vi "mein_sensor.vi"(11 "Position":dbl format="%_3g") -> (3 "Sensorsignal":dbl format="%_3g")   [LabVIEW 2019]
panel:
  out "R_aussen":bool
  out "R":bool
  out "L":bool
  out "L_aussen":bool
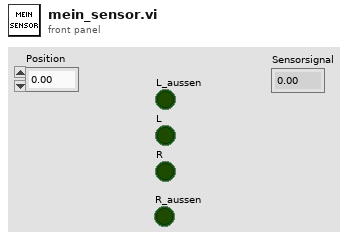
[diagram p1: front panel]
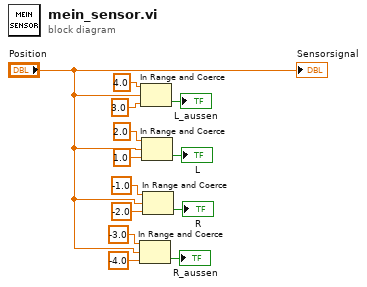
[diagram p0: block diagram]
diagram:
  n1 = In Range and Coerce(upper limit=-3.0, x="Position", lower limit=-4.0) -> (In Range?=→"R_aussen":bool)  [unwired: 1 out]
  n2 = In Range and Coerce(upper limit=4.0, x="Position", lower limit=3.0) -> (In Range?=→"L_aussen":bool)  [unwired: 1 out]
  n3 = In Range and Coerce(upper limit=2.0, x="Position", lower limit=1.0) -> (In Range?=→"L":bool)  [unwired: 1 out]
  n4 = In Range and Coerce(upper limit=-1.0, x="Position", lower limit=-2.0) -> (In Range?=→"R":bool)  [unwired: 1 out]
  "Sensorsignal" <- "Position"
